vi "KalmanFilterLatencyComp_ApplyPastGlobalMeasurement_UKF.vi"(4 "KALMAN_FILTER_LATENCY_COMP_FUNC_GROUP":T5, 6 "NominalDt_Sec":dbl, 7 "Rows":i32, 8 "TimeStamp_Sec":dbl, 9 "Y":T4, 10 "in UNSCENTED_KALMAN_FILTER":T7, 11 "in KalmanFilterLatencyCompensator":T1) -> (0 "Error":bool, 2 "out UNSCENTED_KALMAN_FILTER":T7, 3 "out KalmanFilterLatencyCompensator":T1)   [LabVIEW 2019, in "Trajectory_Library.lvlib"]
doc: "Add past global measurements (such as from vision)to the estimator. This routine is particular for a system that uses an Unscented Kalman FIlter.\n \nInputs: \n - rows -- The rows in the global measurement vector.\n - KalmanLatencyComp -- Data cluster\n - Unscented Kalman FIlter -- Data cluster for the unscented kalman filter (observer). This is used to recalculate the estimated position from the newly applied measurements.\n - y -- The measurement.\n - timestampSeconds -- The timestamp of the measurement.\n - nominalDtSeconds -- The nominal timestep.\n - KALMAN_FILTER_LATENCY_COMP_FUNC_GROUP -- The function references that take calls correct() on the observer.\n\nOutputs:\n - outKalmanLatencyComp -- updated data cluster\n - outUnscented Kalman FIlter -- updated cluster for the unscented kalman filter (observer). \n - Error -- Set to TRUE if an error occured."
uses:
  Trajectory_Library.lvlib
  KALMAN_FILTER_LATENCY_COMP.ctl
  OBSERVER_SNAP_LIST_ITEM.ctl
  OBSERVER_SNAPSHOT.ctl
  <vilib>/Analysis/Matrix/Datatypes/RealMatrix.ctl
  UNSCENTED_KALMAN_FILTER.ctl
  MERWE_SCALED_SIGMA_PTS.ctl
  CALLBACK_FUNC_TYPE.ctl
  KALMAN_FILTER_LATENCY_COMP_FUNC_GROUP.ctl
  <vilib>/Analysis/Matrix/NI_Matrix.lvlib
panel:
  # "<Statess,1>"
  # "<States, States>"
  # "<Inputs, 1>"
  # "<Outputs,  1>"
  # "State Estimate <Statess,1>"
  # "<States, States>"
  # "<States, ?>"
  # "<Statess,  States>"
  # "<Outputs, Outputs>"
  # "<?, 1>"
  # "<?, 1>"
  # "State Estimate <Statess,1>"
  # "<States, States>"
  # "<States, ?>"
  # "<Statess,  States>"
  # "<Outputs, Outputs>"
  # "<?, 1>"
  # "<?, 1>"
  # "<Statess,1>"
  # "<States, States>"
  # "<Inputs, 1>"
  # "<Outputs,  1>"
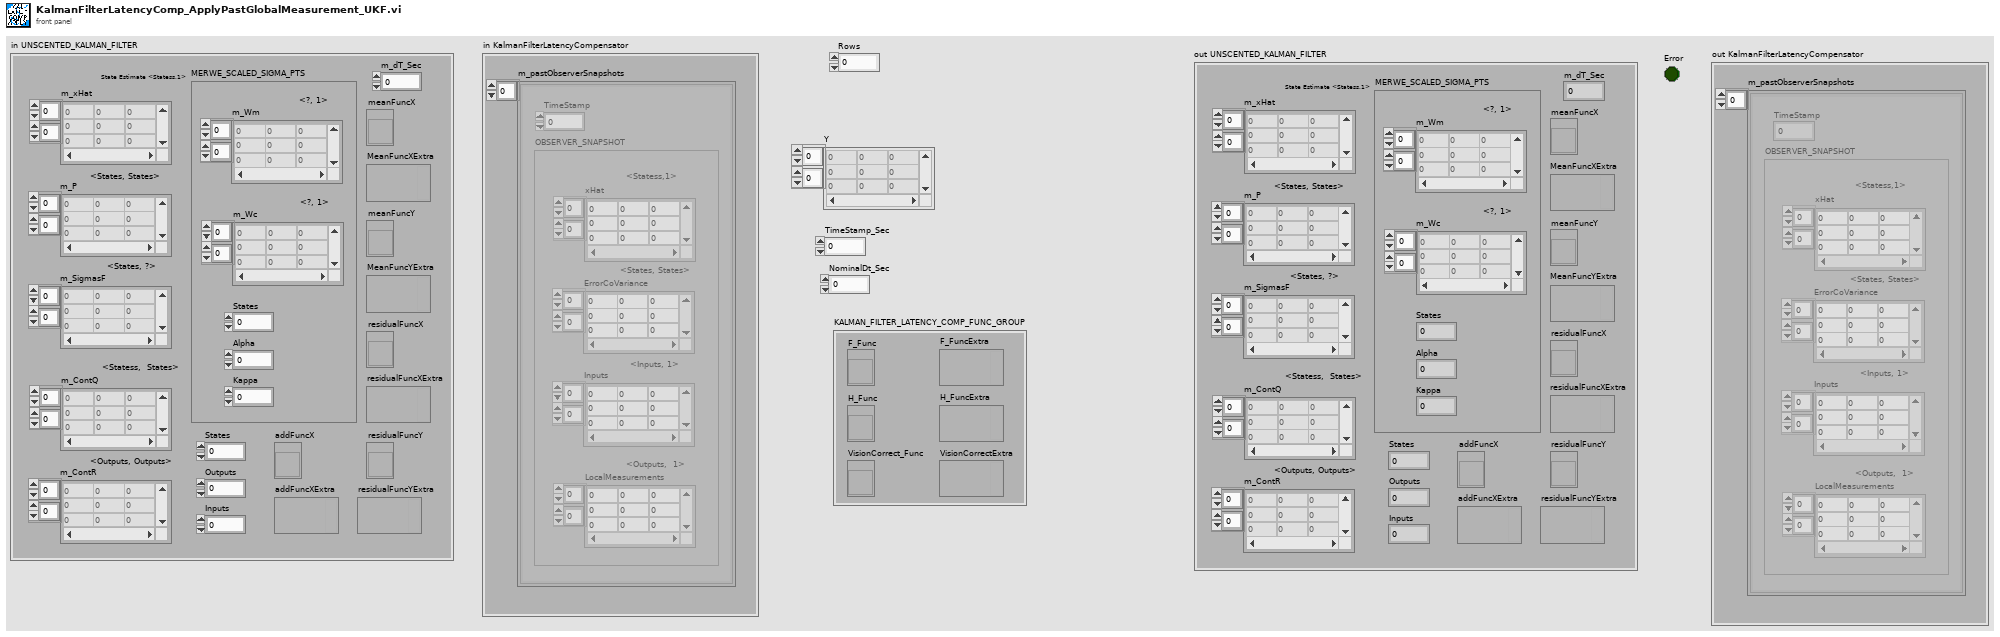
[diagram p1: front panel]
types:
  T1 = typedef "Trajectory_Library.lvlib/KALMAN_FILTER_LATENCY_COMP.ctl" = cluster{"m_pastObserverSnapshots ":T2[]}
  T2 = typedef "Trajectory_Library.lvlib/OBSERVER_SNAP_LIST_ITEM.ctl" = cluster{"TimeStamp":dbl, "OBSERVER_SNAPSHOT":T3}
  T3 = typedef "Trajectory_Library.lvlib/OBSERVER_SNAPSHOT.ctl" = cluster{"ErrorCoVariance":T4, "xHat":T4, "LocalMeasurements":T4, "Inputs":T4}
  T4 = typedef "NI_Matrix.lvlib/RealMatrix.ctl" = dbl[][]
  T5 = typedef "Trajectory_Library.lvlib/KALMAN_FILTER_LATENCY_COMP_FUNC_GROUP.ctl" = cluster{"F_Func":T6, "H_Func":T6, "F_FuncExtra":variant, "H_FuncExtra":variant, "VisionCorrectExtra":variant, "VisionCorrect_Func":refnum<vi>}
  T6 = typedef "Trajectory_Library.lvlib/CALLBACK_FUNC_TYPE.ctl" = refnum<vi>
  T7 = typedef "Trajectory_Library.lvlib/UNSCENTED_KALMAN_FILTER.ctl" = cluster{"m_P":T4, "m_xHat":T4, "States":i32, "Outputs":i32, "m_ContR":T4, "m_ContQ":T4, "m_SigmasF":T4, "m_dT_Sec":dbl, "MERWE_SCALED_SIGMA_PTS":T8, "meanFuncX":T6, "meanFuncY":T6, "residualFuncX":T6, "residualFuncY":T6, "addFuncX":T6, "addFuncXExtra":variant, "residualFuncYExtra":variant, "residualFuncXExtra":variant, "MeanFuncYExtra":variant, "MeanFuncXExtra":variant, "Inputs":i32}
  T8 = typedef "Trajectory_Library.lvlib/MERWE_SCALED_SIGMA_PTS.ctl" = cluster{"m_Wm":T4, "States":i32, "Alpha":dbl, "m_Wc":T4, "Kappa":i32}
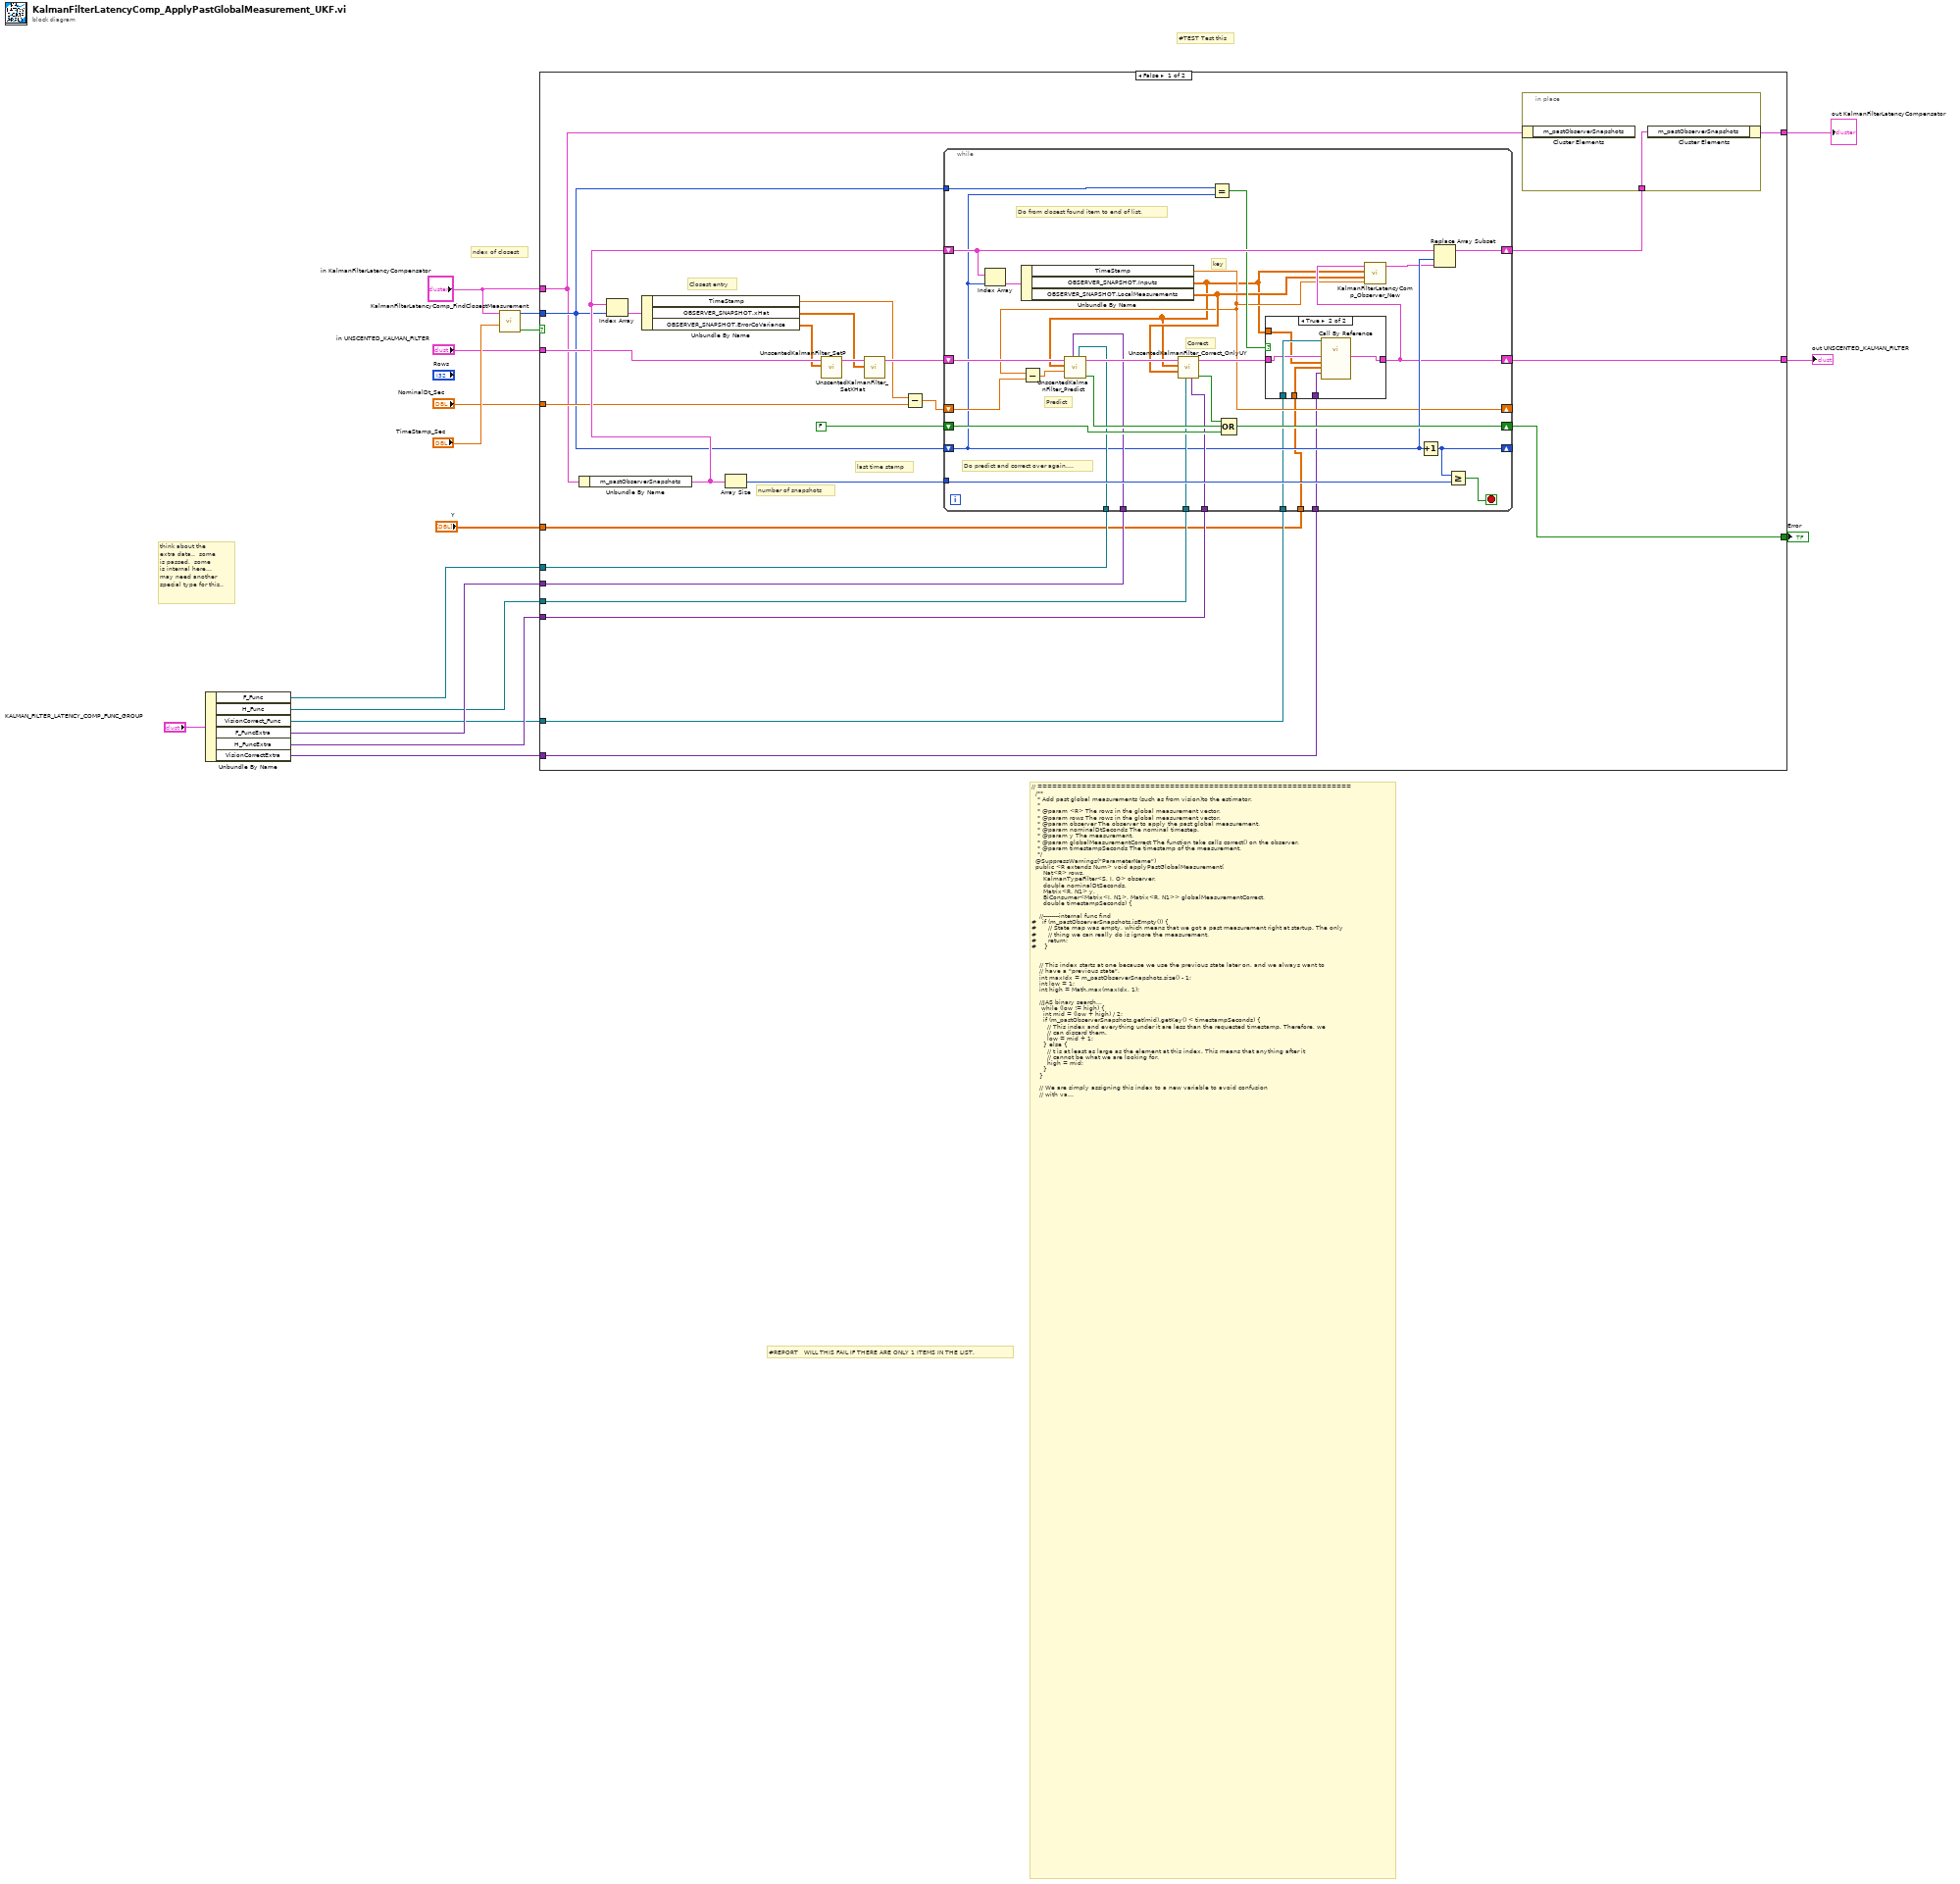
[diagram p0: block diagram]
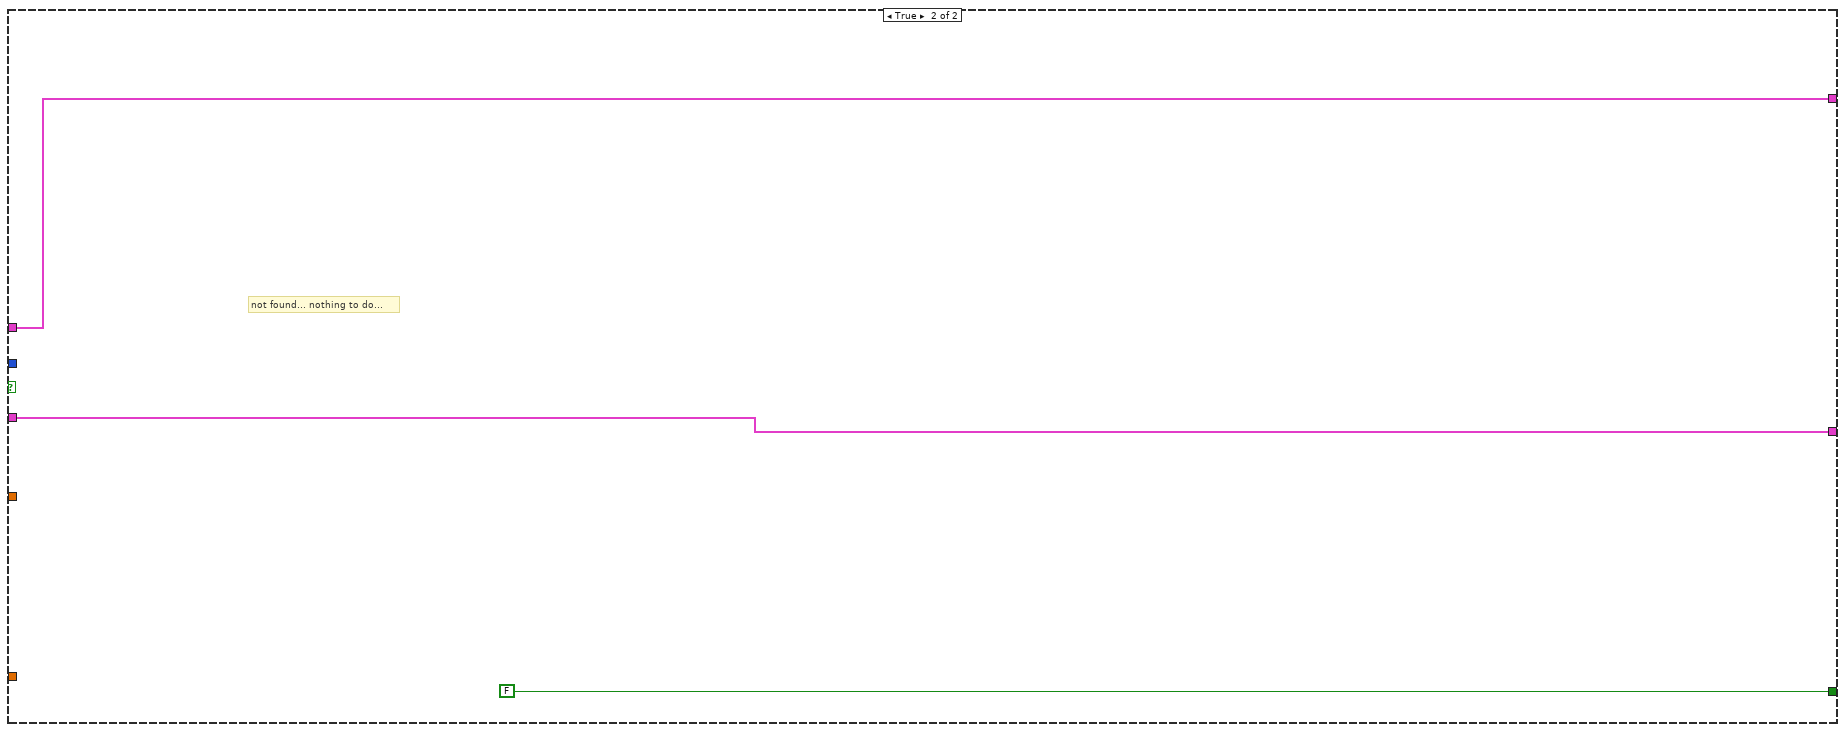
[diagram p3: hidden frame]
diagram:
  # "#TEST Test this"
  # "#REPORT   WILL THIS FAIL IF THERE ARE ONLY 1 ITEMS IN THE LIST."
  # "// ================================================================\n  /**\n   * Add past global measurements (such as from vision)to the estimator.\n   *\n   * @param <R> The rows in the global measurement vector.\n   * @param rows The rows in the global measurement vector.\n   * @param observer The observer to apply the past global measurement.\n   * @param nominalDtSeconds The nominal timestep.\n   * @param y The measurement.\n   * @param globalMeasurementCorrect The function take calls correct() on the observer.\n   * @param timestampSeconds The timestamp of the measurement.\n   */\n  @SuppressWarnings(\"ParameterName\")\n  public <R extends Num> void applyPastGlobalMeasurement(\n      Nat<R> rows,\n      KalmanTypeFilter<S, I, O> observer,\n      double nominalDtSeconds,\n      Matrix<R, N1> y,\n      BiConsumer<Matrix<I, N1>, Matrix<R, N1>> globalMeasurementCorrect,\n      double timestampSeconds) {\n \n    //--------internal func find\n#   if (m_pastObserverSnapshots.isEmpty()) {\n#      // State map was empty, which means that we got a past measurement right at startup. The only\n#      // thing we can really do is ignore the measurement.\n#      return;\n#    }\n\n\n    // This index starts at one because we use the previous state later on, and we always want to\n    // have a \"previous state\".\n    int maxIdx = m_pastObserverSnapshots.size() - 1;\n    int low = 1;\n    int high = Math.max(maxIdx, 1);\n\n    //JAS binary search...\n     while (low != high) {\n      int mid = (low + high) / 2;\n      if (m_pastObserverSnapshots.get(mid).getKey() < timestampSeconds) {\n        // This index and everything under it are less than the requested timestamp. Therefore, we\n        // can discard them.\n        low = mid + 1;\n      } else {\n        // t is at least as large as the element at this index. This means that anything after it\n        // cannot be what we are looking for.\n        high = mid;\n      }\n    }\n\n    // We are simply assigning this index to a new variable to avoid confusion\n    // with variable names.\n    int index = low;\n\n    double timestamp = timestampSeconds;\n\n    // WILL THIS FAIL IF THERE ARE ONLY 1 ITEMS IN THE LIST.\n\n    int indexOfClosestEntry =\n        Math.abs(timestamp - m_pastObserverSnapshots.get(index - 1).getKey())\n                <= Math.abs(\n                    timestamp - m_pastObserverSnapshots.get(Math.min(index, maxIdx)).getKey())\n            ? index - 1\n            : index;\n\n    //--------end of internal func find\n\n    double lastTimestamp =\n        m_pastObserverSnapshots.get(indexOfClosestEntry).getKey() - nominalDtSeconds;\n\n\n\n    // We will now go back in time to the state of the system at the time when\n    // the measurement was captured. We will reset the observer to that state,\n    // and apply correction based on the measurement. Then, we will go back\n    // through all observer states until the present and apply past inputs to\n    // get the present estimated state.\n    for (int i = indexOfClosestEntry; i < m_pastObserverSnapshots.size(); i++) {\n\n      var key = m_pastObserverSnapshots.get(i).getKey();\n      var snapshot = m_pastObserverSnapshots.get(i).getValue();\n\n      if (i == indexOfClosestEntry) {\n        observer.setP(snapshot.errorCovariances);\n        observer.setXhat(snapshot.xHat);\n      }\n\n      observer.predict(snapshot.inputs, key - lastTimestamp);\n      observer.correct(snapshot.inputs, snapshot.localMeasurements);\n\n      if (i == indexOfClosestEntry) {\n        // Note that the measurement is at a timestep close but probably not exactly equal to the\n        // timestep for which we called predict.\n        // This makes the assumption that the dt is small enough that the difference between the\n        // measurement time and the time that the inputs were captured at is very small.\n        globalMeasurementCorrect.accept(snapshot.inputs, y);\n      }\n\n      lastTimestamp = key;\n\n      m_pastObserverSnapshots.set(\n          i,\n          Map.entry(\n              key, new ObserverSnapshot(observer, snapshot.inputs, snapshot.localMeasurements)));\n\n    }  // END OF LOOP\n  }"
  # "ndex of closest"
  # "think about the\nextra data..  some\nis passed.  some\nis internal here...\nmay need another\nspecial type for this.."
  n1 = Unbundle By Name("KALMAN_FILTER_LATENCY_COMP_FUNC_GROUP") -> ("F_Func"=w7:T6, "H_Func"=w5:T6, "VisionCorrect_Func"=w3:refnum<vi>, "F_FuncExtra"=w8:variant, "H_FuncExtra"=w6:variant, "VisionCorrectExtra"=w1:variant)
  n2 = call "KalmanFilterLatencyComp_FindClosestMeasurement.vi"("TimeStamp_Sec"="TimeStamp_Sec", "in KalmanFilterLatencyCompensator"="in KalmanFilterLatencyCompensator") -> ("NotFound"=w16:bool, "Index"=w11:i32)  [unwired: 8 in]
  n3 = case shown="False" w16 {
    tunnel: "in UNSCENTED_KALMAN_FILTER" -> [w39 w83]
    tunnel: [w32 w83] -> w14
    tunnel: "in KalmanFilterLatencyCompensator" -> [w23 w81]
    tunnel: [w30 FALSE] -> w12
    tunnel: w11 -> [w24 _]
    tunnel: "NominalDt_Sec" -> [w35 _]
    tunnel: w8 -> [w29 _]
    tunnel: w7 -> [w28 _]
    tunnel: w5 -> [w27 _]
    tunnel: w6 -> [w26 _]
    tunnel: [w22 w81] -> w4
    tunnel: w3 -> [w20 _]
    tunnel: "Y" -> [w19 _]
    tunnel: w1 -> [w18 _]
    frame False {
      # "number of snapshots"
      # "Closest entry"
      # "last time stamp"
      n4 = Unbundle By Name(w23) -> ("m_pastObserverSnapshots"=w41:T2[])
      n5 = Index Array(array=w41, index=w24) -> (element=w40:T2)
      n6 = Unbundle By Name(w40) -> ("TimeStamp"=w34:dbl, "OBSERVER_SNAPSHOT.xHat"=w36:T4, "OBSERVER_SNAPSHOT.ErrorCoVariance"=w25:T4)
      n7 = Array Size(array=w41) -> (size(s)=w42:i32)
      n8 = call "UnscentedKalmanFilter_SetP.vi"("P"=w25, "in UnscentedKalmanFiilter"=w39) -> ("out UnscentedKalmanFiilter"=w38:T7)  [unwired: 8 in, 1 out]
      n9 = call "UnscentedKalmanFilter_SetXHat.vi"("xHat"=w36, "in UnscentedKalmanFiilter"=w38) -> ("out UnscentedKalmanFiilter"=w37:T7)  [unwired: 8 in, 1 out]
      n10 = Subtract(x=w34, y=w35) -> (x-y=w33:dbl)
      n11 = while {
        shift-right: [w73] -> _
        shift-left: w24 -> [w54]
        tunnel: w42 -> [w72]
        shift-right: [w48] -> _
        shift-left: w33 -> [w67]
        shift-right: [w50] -> w32
        shift-left: w37 -> [w70]
        shift-right: [w62] -> w30
        shift-left: FALSE -> [w65]
        tunnel: w29 -> [w61]
        tunnel: w26 -> [w60]
        tunnel: w28 -> [w59]
        tunnel: w27 -> [w58]
        tunnel: w24 -> [w57]
        shift-right: [w55] -> w21
        shift-left: w41 -> [w56]
        tunnel: w20 -> [w47]
        tunnel: w19 -> [w45]
        tunnel: w18 -> [w44]
        stop <- w71 stop-if-true
        # "key"
        # "Do from closest found item to end of list."
        # "Correct"
        # "Predict"
        # "Do predict and correct over again...."
        n12 = Index Array(array=w56, index=w54) -> (element=w69:T2)
        n13 = Unbundle By Name(w69) -> ("TimeStamp"=w48:dbl, "OBSERVER_SNAPSHOT.Inputs"=w46:T4, "OBSERVER_SNAPSHOT.LocalMeasurements"=w49:T4)
        n14 = Subtract(x=w48, y=w67) -> (x-y=w68:dbl)
        n15 = call "UnscentedKalmanFilter_Predict.vi"("f_Func"=w59, "F_Func_ExtraData"=w61, "dT_Seconds"=w68, "U"=w46, "in UnscentedKalmanFiilter"=w70) -> ("Error"=w64:bool, "out UnscentedKalmanFiilter"=w66:T7)  [unwired: 5 in]
        n16 = call "UnscentedKalmanFilter_Correct_OnlyUY.vi"("H_ExtraData"=w60, "H"=w58, "Y"=w49, "U"=w46, "in UnscentedKalmanFiilter"=w66) -> ("Error"=w63:bool, "out UnscentedKalmanFiilter"=w52:T7)  [unwired: 5 in]
        n17 = Equal?(x=w57, y=w54) -> (x = y?=w53:bool)
        n18 = Compound Arithmetic op=OR(w63, w64, w65) -> (w62:bool)
        n19 = case shown="True" w53 {
          tunnel: w52 -> [w74 w78]
          tunnel: [w74 w79] -> w50
          tunnel: w47 -> [_ w80]
          tunnel: w46 -> [_ w76]
          tunnel: w45 -> [_ w77]
          tunnel: w44 -> [_ w75]
          frame False {
          }
          frame True {
            n20 = call-by-ref "?"(reference=w80, "ExtraPassedData"=w75, "Y"=w77, "U"=w76, "in UNSCENTED_KALMAN_FILTER"=w78) -> ("out UNSCENTED_KALMAN_FILTER"=w79:T7)  [unwired: 7 in, 3 out]
          }
        }
        n21 = call "KalmanFilterLatencyComp_Observer_New.vi"("TimeStamp_Sec"=w48, "LocalY"=w49, "U"=w46, "Observer"=w50) -> ("OBSERVER_LIST_ITEM"=w51:T2)  [unwired: 7 in]
        n22 = Increment(x=w54) -> (x+1=w73:i32)
        n23 = Replace Array Subset(array=w56, new element=w51, index=w54) -> (w55:T2[])
        n24 = Greater Or Equal?(x=w73, y=w72) -> (x >= y?=w71:bool)
      }
      n25 = in-place {
        in-place-border: w21 -> [w43]
        n26 = in-place-cluster #1(w23) -> ()  [unwired: 1 out]
        n27 = in-place-cluster #1("m_pastObserverSnapshots"=w43) -> (w22:T1)
      }
    }
    frame True {
      # "not found... nothing to do..."
    }
  }
  "Error" <- w12
  "out UNSCENTED_KALMAN_FILTER" <- w14
  "out KalmanFilterLatencyCompensator" <- w4
